vi "get_js_fr_gh.vi"(10 "gonghao":string) -> (0 "error 2":errorcluster caption="error out 10", 2 "juese":string)   [LabVIEW 2017, in "Lib_code.lvlib"]
uses:
  Lib_code.lvlib
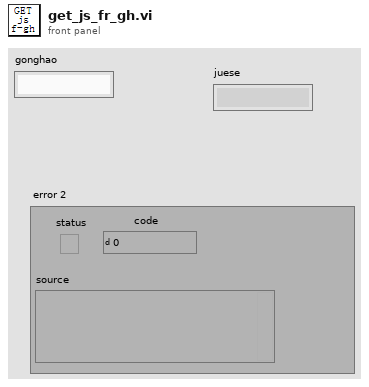
[diagram p1: front panel]
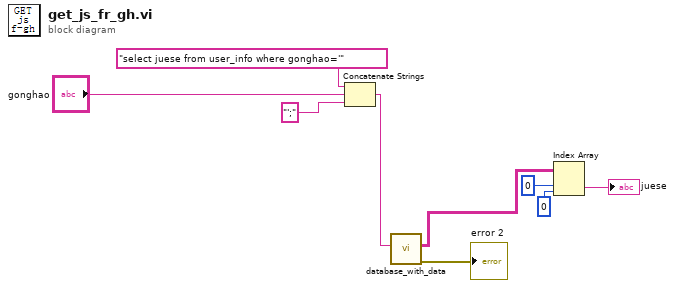
[diagram p0: block diagram]
diagram:
  n1 = Concatenate Strings("select juese from user_info where gonghao='" ("Command Text"), "gonghao", "';" ("字符串")) -> (w6:string)
  n2 = call "database_with_data.vi"("input"=w6) -> ("error"=→"error 2":errorcluster, "Data"=w1:string[][])  [unwired: 9 in]
  n3 = Index Array(array=w1, index (row)=0 ("索引 (行)"), index (col)=0 ("禁用的索引 (列)")) -> (element=→"juese":string)
